vi "copy overides.vi"(7 "application reference (local)":refnum<vi>, 8 "error in":errorcluster, 9 "New class path":path, 10 "New path":path, 11 "Old Path":path) -> (0 "error out":errorcluster)   [LabVIEW 2014, in "FixedChannelTBModuleDecideFeatures.lvclass"]
uses:
  FixedChannelTBModuleDecideFeatures.lvclass
  <vilib>/Utility/traverseref.llb/TRef TravTarget.ctl
  <vilib>/Utility/traverseref.llb/VI Scripting - Traverse.lvlib
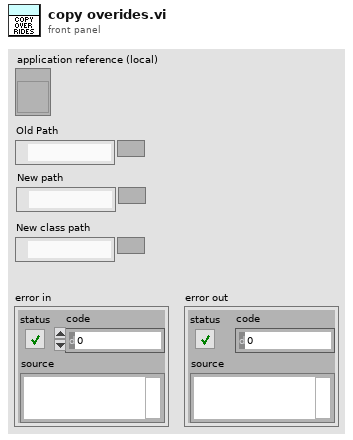
[diagram p1: front panel]
types:
  T1 = typedef "TRef TravTarget.ctl" = enum16{"FP", "BD", "Other"}
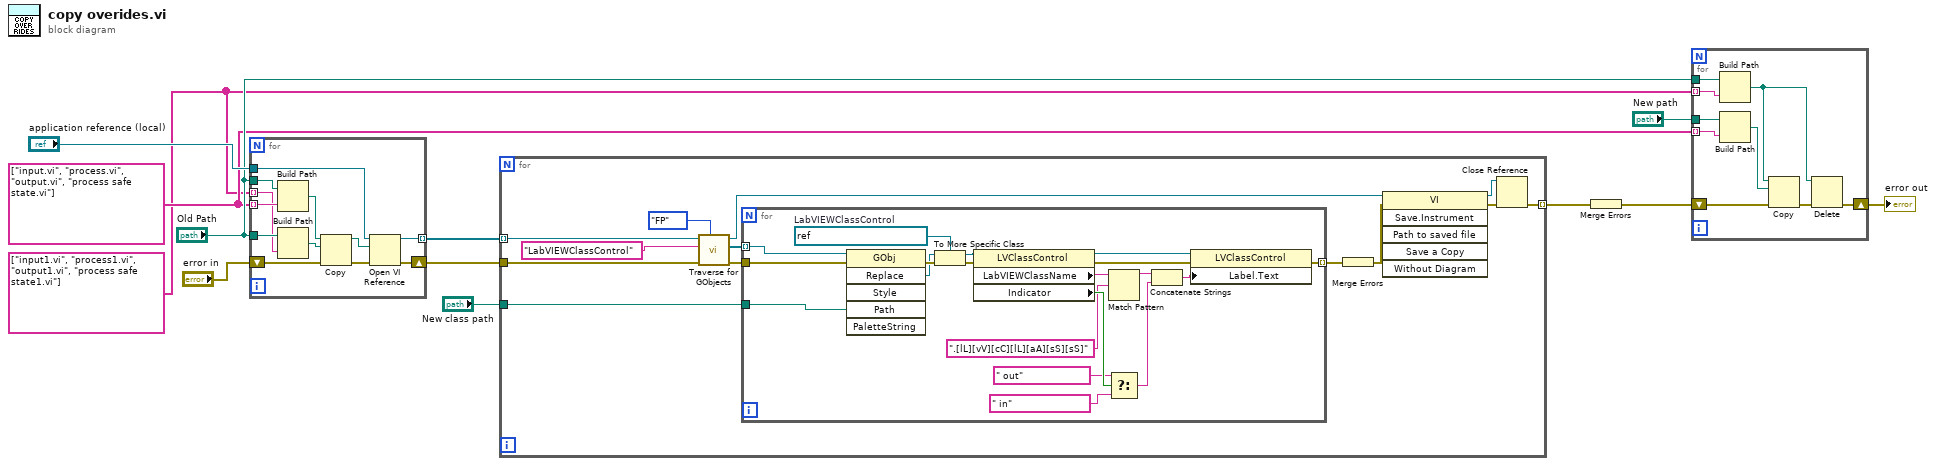
[diagram p0: block diagram]
diagram:
  w1 = string[] ["input1.vi", "process1.vi", "output1.vi", "process safe state1.vi"]
  w5 = string[] ["input.vi", "process.vi", "output.vi", "process safe state.vi"]
  n1 = for {
    tunnel: w5 -> [w22] mode=indexing
    tunnel: "Old Path" -> [w24]
    tunnel: "Old Path" -> [w23]
    shift-right: [w15] -> w10
    shift-left: "error in" -> [w19]
    tunnel: "application reference (local)" -> [w16]
    tunnel: [w14] -> w8 mode=indexing
    tunnel: w1 -> [w13] mode=indexing
    n2 = Build Path(base path=w24, name or relative path=w22) -> (appended path=w21:path)
    n3 = Build Path(base path=w23, name or relative path=w13) -> (appended path=w20:path)
    n4 = Copy(8:w19, 10:w20, 11:w21) -> (0:w18:errorcluster, 3:w17:path)  [unwired: 2 in, 1 out]
    n5 = Open VI Reference(application reference (local)=w16, vi path=w17, error in (no error)=w18) -> (vi reference=w14:refnum<vi>, error out=w15:errorcluster)  [unwired: 3 in]
  }
  n6 = for {
    tunnel: "New class path" -> [w33]
    tunnel: w10 -> [w32]
    tunnel: w8 -> [w31] mode=indexing
    tunnel: [w26] -> w7 mode=indexing
    n7 = call <vilib>:"Traverse for GObjects.vi"("Traverse Target"=TRef_TravTarget."FP", "error in (no error)"=w32, "Class Name"="LabVIEWClassControl", "VI Refnum"=w31) -> ("error out"=w34:errorcluster, "References"=w35:refnum<vi>[], "dup VI Refnum"=w30:refnum<vi>)  [unwired: 4 in, 1 out]
    n8 = for {
      tunnel: w35 -> [w42] mode=indexing
      tunnel: [w43] -> w29 mode=indexing
      tunnel: w33 -> [w41]
      tunnel: w34 -> [w39]
      w54 = refnum<vi> refnum  # LabVIEWClassControl
      n9 = invoke class="GObj" method="Replace"(reference=w42, error in=w39, "Path"=w41) -> (error out=w40:errorcluster, "Replace"=w38:refnum<vi>)  [unwired: 3 in, 4 out]
      n10 = To More Specific Class(target class=w54, reference=w38, error in=w40) -> (specific class reference=w55:refnum<vi>, error out=w56:errorcluster)
      n11 = property class="LVClassControl"(reference=w55, error in=w56) -> (reference out=w53:refnum<vi>, error out=w52:errorcluster, "LabVIEWClassName"=w46:string, "Indicator"=w50:bool)
      n12 = Match Pattern(string=w46, regular expression=".[lL][vV][cC][lL][aA][sS][sS]") -> (before substring=w44:string)  [unwired: 1 in, 3 out]
      n13 = Select(t=" out", s=w50, f=" in") -> (s? t:f=w47:string)
      n14 = Concatenate Strings(w44, w47) -> (w51:string)
      n15 = property class="LVClassControl"(reference=w53, error in=w52, "Label.Text"=w51) -> (error out=w43:errorcluster)  [unwired: 1 out]
    }
    n16 = Merge Errors(w29) -> (w28:errorcluster)
    n17 = invoke class="VI" method="Save.Instrument"(reference=w30, error in=w28) -> (reference out=w25:refnum<vi>, error out=w27:errorcluster)  [unwired: 4 in, 4 out]
    n18 = Close Reference(reference=w25, error in (no error)=w27) -> (error out=w26:errorcluster)
  }
  n19 = Merge Errors(w7) -> (w3:errorcluster)
  n20 = for {
    tunnel: w1 -> [w63] mode=indexing
    tunnel: "Old Path" -> [w65]
    tunnel: "New path" -> [w64]
    shift-right: [w57] -> w2
    shift-left: w3 -> [w61]
    tunnel: w5 -> [w60] mode=indexing
    n21 = Build Path(base path=w65, name or relative path=w63) -> (appended path=w58:path)
    n22 = Build Path(base path=w64, name or relative path=w60) -> (appended path=w62:path)
    n23 = Copy(8:w61, 10:w62, 11:w58) -> (0:w59:errorcluster)  [unwired: 2 in, 2 out]
    n24 = Delete(path (use dialog)=w58, error in=w59) -> (error out=w57:errorcluster)  [unwired: 3 in, 2 out]
  }
  "error out" <- w2
